vi "ReadWriteTopicData.vi"(3 "error in (no error)":errorcluster, 4 "timeout ms (1000)":i32=1000, 5 "connection ID in":refnum<k5>) -> (0 "error out":errorcluster, 1 "data out":string, 2 "connection ID out":refnum<k5>)   [LabVIEW 2012]
doc: "Reads and writes topic data"
uses:
  <userlib>/ROSforLV/ROS/parsing/std_msgs/subs/parse_u32_scalar.vi
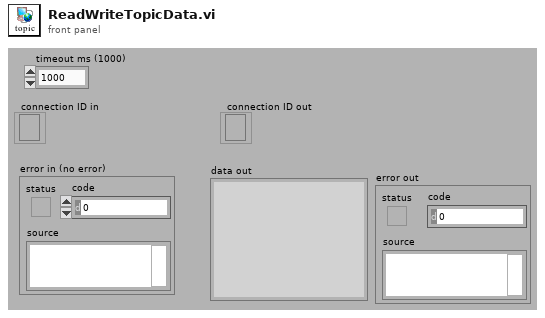
[diagram p1: front panel]
types:
  T1 = enum16{"Standard", "Buffered", "CRLF", "Immediate"}
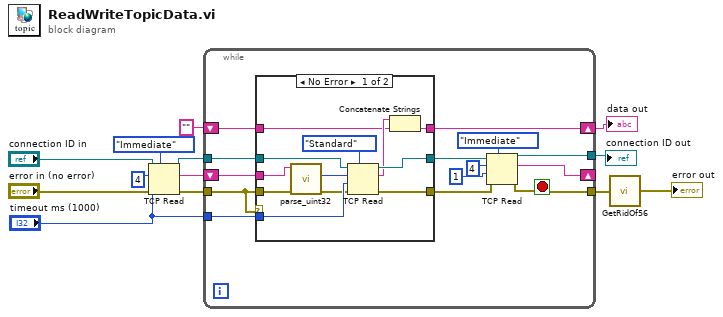
[diagram p0: block diagram]
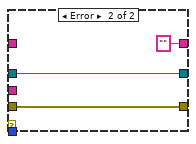
[diagram p2: hidden frame]
diagram:
  n1 = TCP Read(connection ID="connection ID in", bytes to read=4, error in (no error)="error in (no error)", 7:T1."Immediate" ("mode (standard)"), 9:"timeout ms (1000)") -> (connection ID out=w9:refnum<k5>, data out=w6:string, error out=w5:errorcluster)
  n2 = while {
    tunnel: [w14] -> w12
    tunnel: w9 -> [w26]
    tunnel: w5 -> [w24]
    tunnel: "timeout ms (1000)" -> [w23]
    tunnel: [w19] -> w3
    shift-right: [w17] -> _
    shift-left: w6 -> [w25]
    shift-right: [w27] -> w13
    shift-left: "" ("data out") -> [w15]
    stop <- w14 stop-if-true
    n3 = case shown="No Error" w24 {
      tunnel: [w28 "" ("data out")] -> w27
      tunnel: [w39 w41] -> w18
      tunnel: [w38 w42] -> w22
      tunnel: w24 -> [w33 w41]
      tunnel: w26 -> [w37 w42]
      tunnel: w25 -> [w31 _]
      tunnel: w23 -> [w35 _]
      tunnel: w15 -> [w29 _]
      frame No Error {
        n4 = call-poly <userlib>:"parse_uint32.vi"("error in"=w33, "msg in"=w31) -> ("error out"=w32:errorcluster, "number"=w34:u32)  [unwired: 3 in, 1 out]
        n5 = TCP Read(connection ID=w37, bytes to read=w34, error in (no error)=w32, 7:T1."Standard" ("mode (standard)"), 9:w35) -> (connection ID out=w38:refnum<k5>, data out=w30:string, error out=w39:errorcluster)
        n6 = Concatenate Strings(w30, w29) -> (w28:string)
      }
      frame Error {
      }
    }
    n7 = TCP Read(connection ID=w22, bytes to read=4, error in (no error)=w18, 7:T1."Immediate" ("mode (standard)"), 9:1 ("timeout ms (25000)")) -> (connection ID out=w19:refnum<k5>, data out=w17:string, error out=w14:errorcluster)
  }
  "data out" <- w13
  "connection ID out" <- w3
  n8 = call <userlib>:"GetRidOf56.vi"("error in (no error)"=w12) -> ("error out"=→"error out":errorcluster)
